vi "RAMP_write_laser_line_item_name.vi"(2 "Laser line number":i32, 3 "Laser application":i32, 4 "Power or time":i32, 5 "Laser line":i32) -> (1 "Item name":string)   [LabVIEW 2015]
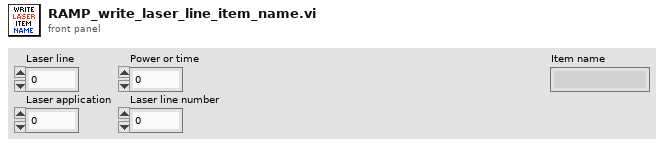
[diagram p1: front panel]
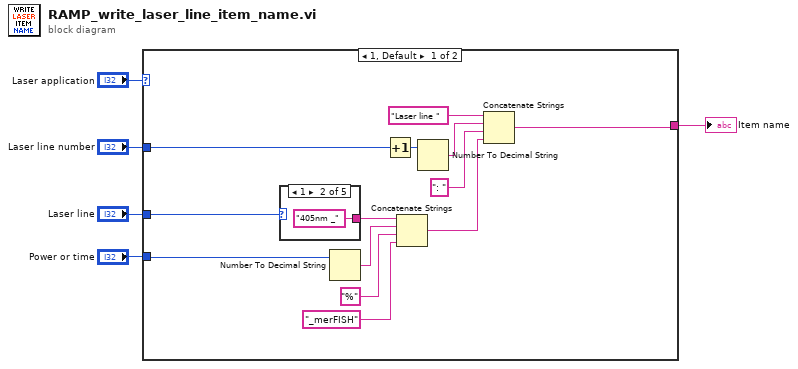
[diagram p0: block diagram]
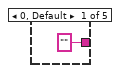
[diagram p2: hidden frame]
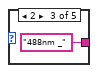
[diagram p3: hidden frame]
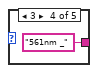
[diagram p4: hidden frame]
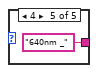
[diagram p5: hidden frame]
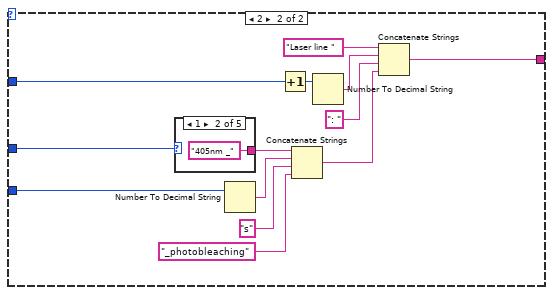
[diagram p6: hidden frame]
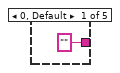
[diagram p7: hidden frame]
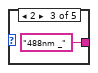
[diagram p8: hidden frame]
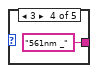
[diagram p9: hidden frame]
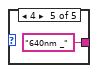
[diagram p10: hidden frame]
diagram:
  n1 = case shown="1, Default" "Laser application" {
    tunnel: "Laser line" -> [w8 w27]
    tunnel: [w9 w26] -> w3
    tunnel: "Laser line number" -> [w7 w25]
    tunnel: "Power or time" -> [w6 w24]
    frame 1, Default {
      n2 = case shown="1" w8 {
        tunnel: ["" "405nm _" "488nm _" "561nm _" "640nm _"] -> w14
        frame 0, Default {
        }
        frame 1 {
        }
        frame 2 {
        }
        frame 3 {
        }
        frame 4 {
        }
      }
      n3 = Number To Decimal String(number=w6) -> (decimal integer string=w15:string)  [unwired: 1 in]
      n4 = Increment(x=w7) -> (x+1=w11:i32)
      n5 = Concatenate Strings(w14, w15, "%" ("string"), "_merFISH") -> (w17:string)
      n6 = Number To Decimal String(number=w11) -> (decimal integer string=w12:string)  [unwired: 1 in]
      n7 = Concatenate Strings("Laser line " ("string"), w12, ": " ("string"), w17) -> (w9:string)
    }
    frame 2 {
      n8 = case shown="1" w27 {
        tunnel: ["" "405nm _" "488nm _" "561nm _" "640nm _"] -> w32
        frame 0, Default {
        }
        frame 1 {
        }
        frame 2 {
        }
        frame 3 {
        }
        frame 4 {
        }
      }
      n9 = Number To Decimal String(number=w24) -> (decimal integer string=w33:string)  [unwired: 1 in]
      n10 = Increment(x=w25) -> (x+1=w29:i32)
      n11 = Concatenate Strings(w32, w33, "s" ("string"), "_photobleaching") -> (w35:string)
      n12 = Number To Decimal String(number=w29) -> (decimal integer string=w30:string)  [unwired: 1 in]
      n13 = Concatenate Strings("Laser line " ("string"), w30, ": " ("string"), w35) -> (w26:string)
    }
  }
  "Item name" <- w3
